vi "_Get Meas Error Codes.vi"(8 "error in (no error)":errorcluster, 10 "Command":string, 11 "VISA resource name":refnum<visa-resource-name>) -> (0 "error out":errorcluster, 1 "Reliability":i32, 2 "Error Codes":i32[](array[numeric]), 3 "VISA resource name out":refnum<visa-resource-name>)   [LabVIEW 2020, in "Rohde&Schwarz CMXP GPRF.lvlib"]
uses:
  <instrlib>/Rohde&Schwarz CMXP GPRF/Rohde&Schwarz CMXP GPRF.lvlib
  <instrlib>/Rohde&Schwarz CMXP GPRF/Private/rsidr_core.llb/rsidr_core.lvlib
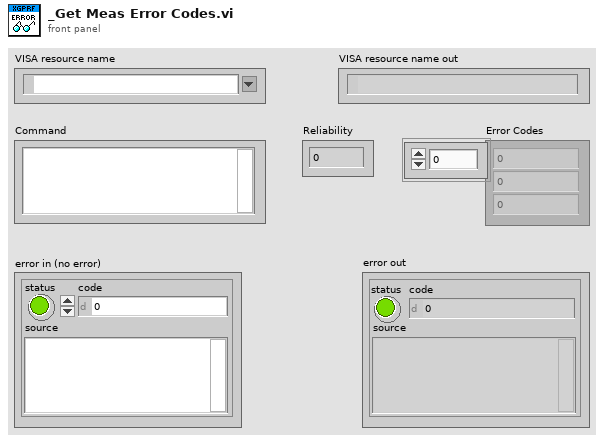
[diagram p1: front panel]
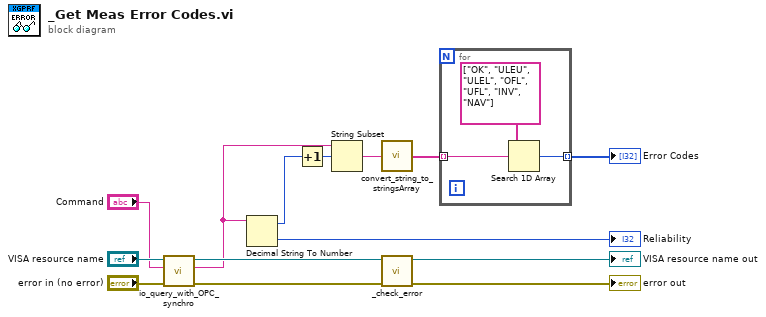
[diagram p0: block diagram]
diagram:
  n1 = call <instrlib>:"io_query_with_OPC_synchro.vi"("error in"="error in (no error)", "write buffer"="Command", "VISA resource name"="VISA resource name") -> ("error out"=w13:errorcluster, "read buffer"=w5:string, "VISA resource name out"=w14:refnum<visa-resource-name>)  [unwired: 6 in]
  n2 = Decimal String To Number(string=w5) -> (offset past number=w7:i32, number=→"Reliability":i32)  [unwired: 2 in]
  n3 = Increment(x=w7) -> (x+1=w8:i32)
  n4 = String Subset(string=w5, offset (0)=w8) -> (substring=w6:string)  [unwired: 1 in]
  n5 = call <instrlib>:"convert_string_to_stringsArray.vi"("String in"=w6) -> ("string array out"=w3:string[])  [unwired: 3 in, 1 out]
  n6 = call <instrlib>:"_check_error.vi"("error in (no error)"=w13, "VISA resource name"=w14) -> ("error out"=→"error out":errorcluster, "VISA resource name out"=→"VISA resource name out":refnum<visa-resource-name>)  [unwired: 8 in]
  n7 = for {
    tunnel: w3 -> [w17] mode=indexing
    tunnel: [w16] -> w2 mode=indexing
    n8 = Search 1D Array(1D array=string[] ["OK", "ULEU", "ULEL", "OFL", "UFL", "INV", "NAV"], element=w17) -> (index of element=w16:i32)  [unwired: 1 in]
  }
  "Error Codes" <- w2
